vi "Find max and min values in X and Y data array.vi"(9 "Function":enum16{"Analyse & store", "Read stored values"}(ring), 11 "Data In":T1) -> (0 "Min time among all datasets":dbl, 1 "Max time among all datasets":dbl, 2 "Min intensity among all datasets":dbl, 3 "Max intensity among all datasets":dbl, 4 "Max number of points":i32)   [LabVIEW 2017, in "XGrapher.xctl"]
uses:
  XGrapher.xctl
  Data 1.ctl
  Typedefs/Xctrl-Data array.ctl
  Typedefs/Xcrtl-Data format definition.ctl
  Typedefs/Xctl-XY data type definition.ctl
  Typedefs/Xctrl-ROI type enum.ctl
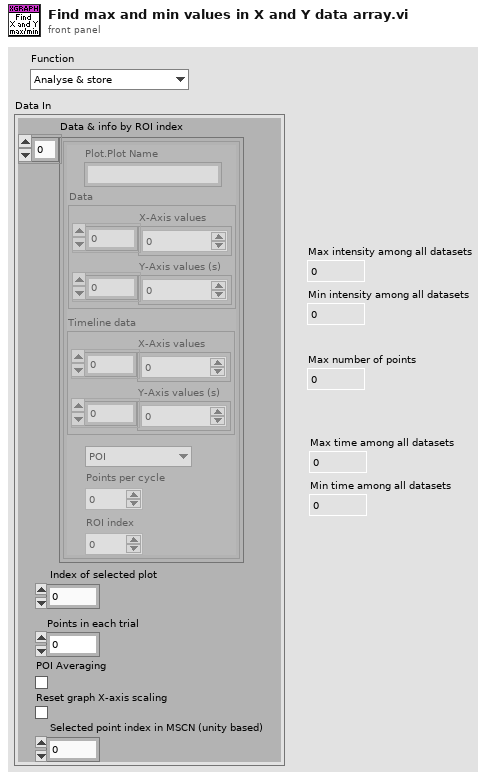
[diagram p1: front panel]
types:
  T1 = typedef "XGrapher.xctl/Data 1.ctl" = cluster{"Data & info by ROI index":T2, "Index of selected plot":u16, "Points in each trial":i32, "POI Averaging":bool, "Reset graph X-axis scaling":bool, "Selected point index in MSCN (unity based)":u16}
  T2 = typedef "Xctrl-Data array.ctl" = T3[]
  T3 = typedef "XGrapher.xctl/Xcrtl-Data format definition.ctl" = cluster{"Plot.Plot Name":string, "Data":T4, "Timeline data":T4, "Type":T5, "Points per cycle":u16, "ROI index":u16}
  T4 = typedef "XGrapher.xctl/Xctl-XY data type definition.ctl" = cluster{"X-Axis values":sgl[], "Y-Axis values (s)":sgl[]}
  T5 = typedef "Xctrl-ROI type enum.ctl" = enum16{"POI", "Mini-scan", "Group"}
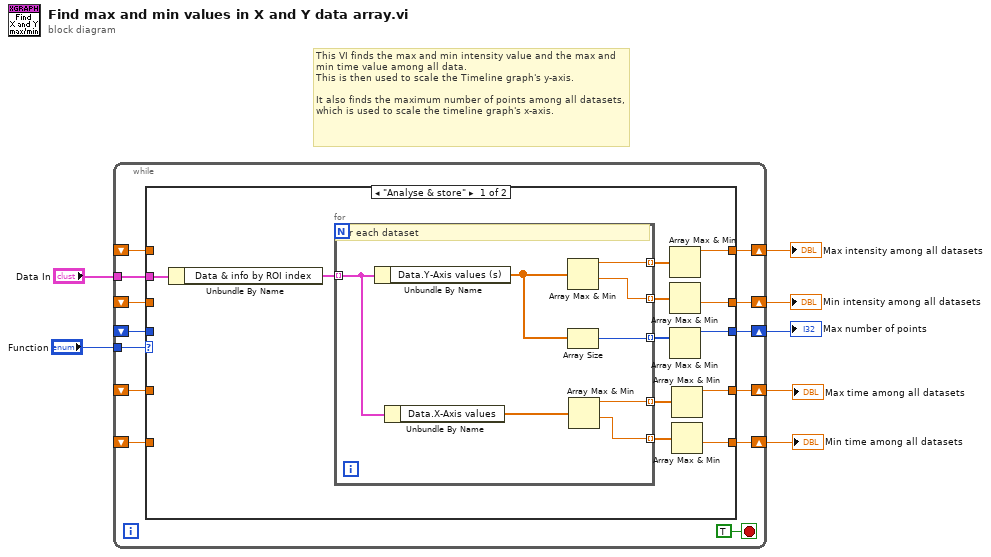
[diagram p0: block diagram]
diagram:
  # "This VI finds the max and min intensity value and the max and min time value among all data.\nThis is then used to scale the Timeline graph's y-axis.\n\nIt also finds the maximum number of points among all datasets, which is used to scale the timeline graph's x-axis."
  n1 = while {
    tunnel: "Data In" -> [w19]
    shift-right: [w15] -> w2
    shift-left: _ -> [w9]
    shift-right: [w17] -> w4
    shift-left: _ -> [w10]
    shift-right: [w18] -> w5
    shift-left: _ -> [w11]
    shift-right: [w16] -> w3
    shift-left: _ -> [w12]
    shift-right: [w20] -> w7
    shift-left: _ -> [w13]
    tunnel: "Function" -> [w8]
    stop <- TRUE stop-if-true
    n2 = case shown="\"Analyse & store\"" w8 {
      tunnel: [w32 w45] -> w20
      tunnel: w19 -> [w30 _]
      tunnel: [w28 w43] -> w18
      tunnel: [w26 w42] -> w17
      tunnel: [w23 w44] -> w16
      tunnel: [w21 w41] -> w15
      tunnel: w13 -> [_ w45]
      tunnel: w12 -> [_ w44]
      tunnel: w11 -> [_ w43]
      tunnel: w10 -> [_ w42]
      tunnel: w9 -> [_ w41]
      frame "Analyse & store" {
        n3 = Unbundle By Name(w30) -> ("Data & info by ROI index"=w31:T2)
        n4 = for {
          tunnel: w31 -> [w39] mode=indexing
          tunnel: [w40] -> w29 mode=indexing
          tunnel: [w34] -> w27 mode=indexing
          tunnel: [w37] -> w25 mode=indexing
          tunnel: [w36] -> w24 mode=indexing
          tunnel: [w33] -> w22 mode=indexing
          # "For each dataset"
          n5 = Unbundle By Name(w39) -> ("Data.Y-Axis values (s)"=w38:sgl[])
          n6 = Unbundle By Name(w39) -> ("Data.X-Axis values"=w35:sgl[])
          n7 = Array Max & Min(array=w38) -> (max value=w37:sgl, min value=w36:sgl)  [unwired: 2 out]
          n8 = Array Size(array=w38) -> (size(s)=w40:i32)
          n9 = Array Max & Min(array=w35) -> (max value=w34:sgl, min value=w33:sgl)  [unwired: 2 out]
        }
        n10 = Array Max & Min(array=w25) -> (max value=w32:sgl)  [unwired: 3 out]
        n11 = Array Max & Min(array=w24) -> (min value=w23:sgl)  [unwired: 3 out]
        n12 = Array Max & Min(array=w29) -> (max value=w28:i32)  [unwired: 3 out]
        n13 = Array Max & Min(array=w27) -> (max value=w26:sgl)  [unwired: 3 out]
        n14 = Array Max & Min(array=w22) -> (min value=w21:sgl)  [unwired: 3 out]
      }
      frame "Read stored values", Default {
      }
    }
  }
  "Max intensity among all datasets" <- w7
  "Min intensity among all datasets" <- w3
  "Max number of points" <- w5
  "Max time among all datasets" <- w4
  "Min time among all datasets" <- w2
